vi "Initial State.vi"(8 "error in (no error)":errorcluster, 10 "Initial State":refnum<class "_State Machine Actor.lvclass">, 11 "Automation Controller in":refnum<class "Automation Controller.lvclass">) -> (0 "error out":errorcluster, 3 "Automation Controller out":refnum<class "Automation Controller.lvclass">)   [LabVIEW 2024, in "Automation Controller.lvlib" / "Automation Controller.lvclass"]
uses:
  Automation Controller.lvclass
  Automation Controller.lvclass/Automation Controller.ctl
  _State Machine Actor/_State Machine Actor/_State Machine Actor.lvclass
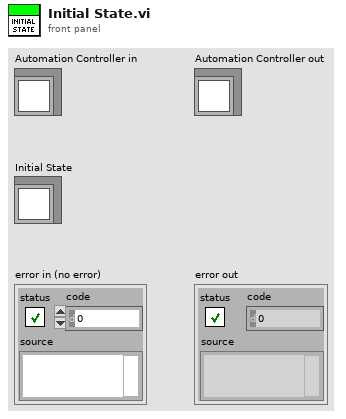
[diagram p1: front panel]
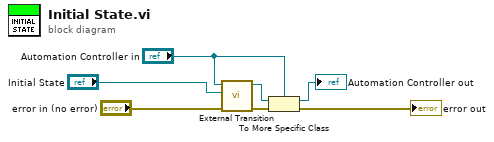
[diagram p0: block diagram]
diagram:
  n1 = call-dynamic "External Transition.vi"("error in (no error)"="error in (no error)", "Target State"="Initial State", "State Machine Actor in"="Automation Controller in") -> ("error out"=w2:errorcluster, "_State Machine Actor out"=w7:refnum<class "_State Machine Actor.lvclass">)  [unwired: 7 in]
  n2 = To More Specific Class(target class="Automation Controller in", reference=w7, error in=w2) -> (specific class reference=→"Automation Controller out":refnum<class "Automation Controller.lvclass">, error out=→"error out":errorcluster)
